vi "shutdown - 2.vi"   [LabVIEW 2015]
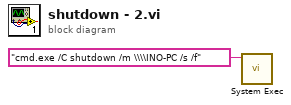
[diagram p0: block diagram]
diagram:
  n1 = call <vilib>:"System Exec.vi"("command line"="cmd.exe /C shutdown /m \\\\INO-PC /s /f") -> ()  [unwired: 7 in, 4 out]
